vi "Main On Compile Action VI.vi"(8 "error in (no error)":errorcluster, 11 "Device Item Ref in":T1 format="%.0x") -> (0 "error out":errorcluster)   [LabVIEW 2015, in "NI 9759 RevB Custom Device.lvlib"]
uses:
  NI 9759 RevB Custom Device.lvlib
  <vilib>/NI Veristand/Custom Device API/Custom Device Item Ref.ctl
  Shared/Types/Compiled Data.ctl
  Shared/Types/RT Init Data.ctl
  Shared/Types/RT Status.ctl
  Shared/Types/9759 RevB.ctl
  Shared/9759 Properties.vi
  <vilib>/NI VeriStand/Custom Device API/Custom Device API.lvlib
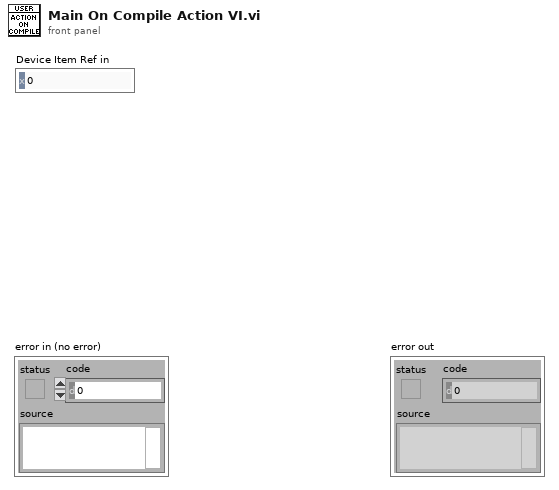
[diagram p1: front panel]
types:
  T1 = typedef "Custom Device API.lvlib/Custom Device Item Ref.ctl" = u64
  T2 = typedef "NI 9759 RevB Custom Device.lvlib/Compiled Data.ctl" = cluster{"DeviceOutFIFO":refnum<k33>, "DeviceInFIFO":refnum<k33>, "Init":T3, "Status":T4, "9759 RevB":T5}
  T3 = typedef "NI 9759 RevB Custom Device.lvlib/RT Init Data.ctl" = cluster{"CPU":i32, "RIO Address":string, "Decimation":i32, "Priority":i32, "Name":string, "Bitfile Path":path, "Input FIFO Size":i32, "Output FIFO Size":i32, "Compile Time":dbl}
  T4 = typedef "NI 9759 RevB Custom Device.lvlib/RT Status.ctl" = cluster{"FIFO indexes":cluster{"code":i32, "loop duration":i32, "late count":i32}}
  T5 = typedef "NI 9759 RevB Custom Device.lvlib/9759 RevB.ctl" = cluster{"FIFO Indexes":cluster{"Read":cluster{"TP1":i32, "TP2":i32, "Analog1":i32, "Analog2":i32, "ISense1":i32, "ISense2":i32, "Battery":i32, "Temperature":i32, "ModulePresent":i32, "Fault1":i32, "Fault2":i32}, "Write":cluster{"ModuleEnable":i32, "ControlEnable1":i32, "ControlEnable2":i32, "Setpoint1":i32, "Setpoint2":i32}}, "Settings":cluster{"PositionCals":cluster{"TPArray (V)":sgl[], "TPArray (deg)":sgl[]}[], "ControlCals":cluster{"TLead (sec)":sgl, "TLag (sec)":sgl, "KRpos (V/deg)":sgl, "TIpos (sec)":sgl, "TDpos (sec)":sgl, "KRneg (V/deg)":sgl, "TIneg (sec)":sgl, "TDneg (sec)":sgl, "ThetaLHErrThresh (deg)":sgl, "ULH (V)":sgl, "ULHLag (sec)":sgl, "US (V)":sgl, "USLag (sec)":sgl, "ThetaLH (deg)":sgl, "MotorResistance (Ohms)":sgl, "BattNom (V)":sgl, "BattCompEnable":bool}[]}}
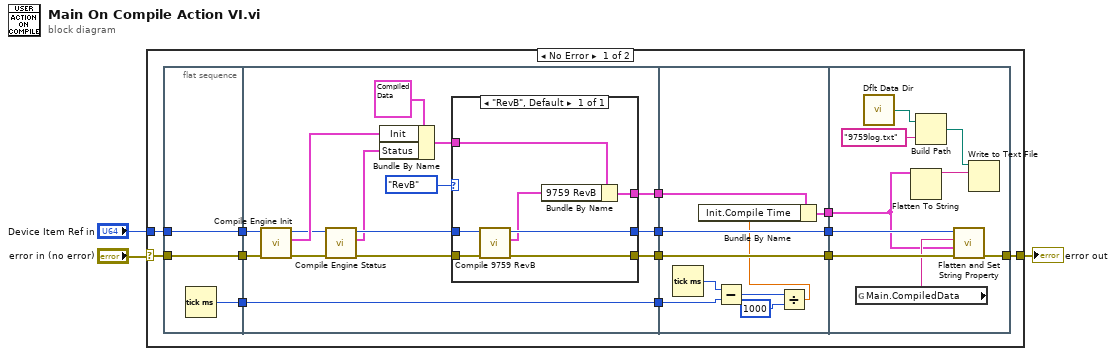
[diagram p0: block diagram]
diagram:
  n1 = case shown="No Error" "error in (no error)" {
    selector: "error in (no error)" -> [w15 w60]
    tunnel: [w11 w60] -> w2
    tunnel: "Device Item Ref in" -> [w16 _]
    frame No Error {
      n2 = flat-sequence {
        tunnel: w15 -> [w18]
        tunnel: w16 -> [w19]
        tunnel: [w19] -> w14
        tunnel: [w18] -> w13
        tunnel: [w17] -> w12
        tunnel: w14 -> [w32]
        tunnel: w13 -> [w31]
        tunnel: w12 -> [w21]
        tunnel: [w24] -> w10
        tunnel: [w23] -> w8
        tunnel: [w22] -> w6
        tunnel: [w21] -> w4
        tunnel: w10 -> [w50]
        tunnel: [w50] -> w9
        tunnel: w8 -> [w49]
        tunnel: [w49] -> w7
        tunnel: w6 -> [w47]
        tunnel: [w48] -> w5
        tunnel: w4 -> [w45]
        tunnel: w9 -> [w58]
        tunnel: w7 -> [w59]
        tunnel: w5 -> [w51]
        tunnel: [w56] -> w11
        frame #0 {
          n3 = Tick Count (ms)() -> (millisecond timer value=w17:u32)
        }
        frame #1 {
          n4 = call "Compile Engine Init.vi"("error in (no error)"=w31, "Device Item Ref in"=w32) -> ("error out"=w25:errorcluster, "System"=w34:T3, "Device Item Ref out"=w26:T1)  [unwired: 7 in]
          n5 = call "Compile Engine Status.vi"("error in (no error)"=w25, "Device Item Ref in"=w26) -> ("error out"=w30:errorcluster, "Status"=w28:T4, "Device Item Ref out"=w29:T1)  [unwired: 7 in]
          n6 = Bundle By Name(cluster=T2 {"DeviceOutFIFO"=refnum, "DeviceInFIFO"=refnum, "Init"={"CPU"=0, "RIO Address"="", "Decimation"=0, "Priority"=0, "Name"="", "Bitfile Path"=path "", "Input FIFO Size"=0, "Output FIFO Size"=0, "Compile Time"=0.0}, "Status"={"FIFO indexes"={"code"=0, "loop duration"=0, "late count"=0}}, "9759 RevB"={"FIFO Indexes"={"Read"={"TP1"=0, "TP2"=0, "Analog1"=0, "Analog2"=0, "ISense1"=0, "ISense2"=0, "Battery"=0, "Temperature"=0, "ModulePresent"=0, "Fault1"=0, "Fault2"=0}, "Write"={"ModuleEnable"=0, "ControlEnable1"=0, "ControlEnable2"=0, "Setpoint1"=0, "Setpoint2"=0}}, "Settings"={"PositionCals"=[], "ControlCals"=[]}}} ("Compiled Data"), "Init"=w34, "Status"=w28) -> (w33:T2)
          n7 = case shown="\"RevB\", Default" enum16{"RevB", "RevB2"}."RevB" ("Version") {
            tunnel: w33 -> [w41]
            tunnel: w30 -> [w36]
            tunnel: w29 -> [w39]
            tunnel: [w37] -> w24
            tunnel: [w38] -> w23
            tunnel: [w40] -> w22
            frame "RevB", Default {
              n8 = call "Compile 9759 RevB.vi"("error in (no error)"=w36, "Device Item Ref in"=w39) -> ("error out"=w37:errorcluster, "9759 RevB"=w35:T5, "Device Item Ref out"=w38:T1)  [unwired: 7 in]
              n9 = Bundle By Name(cluster=w41, "9759 RevB"=w35) -> (w40:T2)
            }
          }
        }
        frame #2 {
          n10 = Tick Count (ms)() -> (millisecond timer value=w46:u32)
          n11 = Subtract(x=w46, y=w45) -> (x-y=w44:u32)
          n12 = Divide(x=w44, y=u32 1000) -> (x/y=w42:dbl)
          n13 = Bundle By Name(cluster=w47, "Init.Compile Time"=w42) -> (w48:T2)
        }
        frame #3 {
          n14 = global read "9759 Properties.vi" "Main.CompiledData"() -> (w57:string)
          n15 = call <vilib>:"Dflt Data Dir.vi"() -> ("App:Default Data Directory"=w54:path)
          n16 = Flatten To String(anything=w51) -> (data string=w55:string)  [unwired: 3 in, 2 out]
          n17 = Build Path(base path=w54, name or relative path="9759log.txt") -> (appended path=w52:path)
          n18 = call "Flatten and Set String Property.vi"("error in (no error)"=w58, "Value"=w51, "Property Name"=w57, "Section Ref in"=w59) -> ("error out"=w56:errorcluster)  [unwired: 6 in, 1 out]
          n19 = Write to Text File(file (use dialog)=w52, text=w55) -> ()  [unwired: 2 in, 3 out]
        }
      }
    }
    frame Error {
    }
  }
  "error out" <- w2
